vi "LinearPos Restrictions.vi"(5 "Robot Width":dbl, 6 "Robot Height":dbl, 7 "Pole Height \n(from ground)":dbl, 8 "Forearm Length":dbl, 9 "Backarm Length":dbl, 10 "newY":dbl, 11 "newX":dbl) -> (2 "modified Y":dbl, 3 "modified X":dbl)   [LabVIEW 2017]
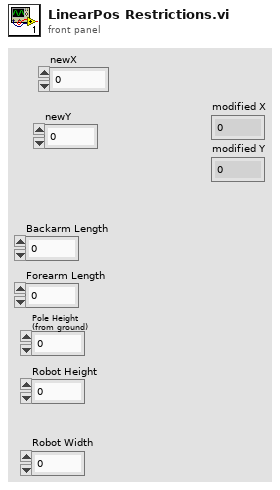
[diagram p1: front panel]
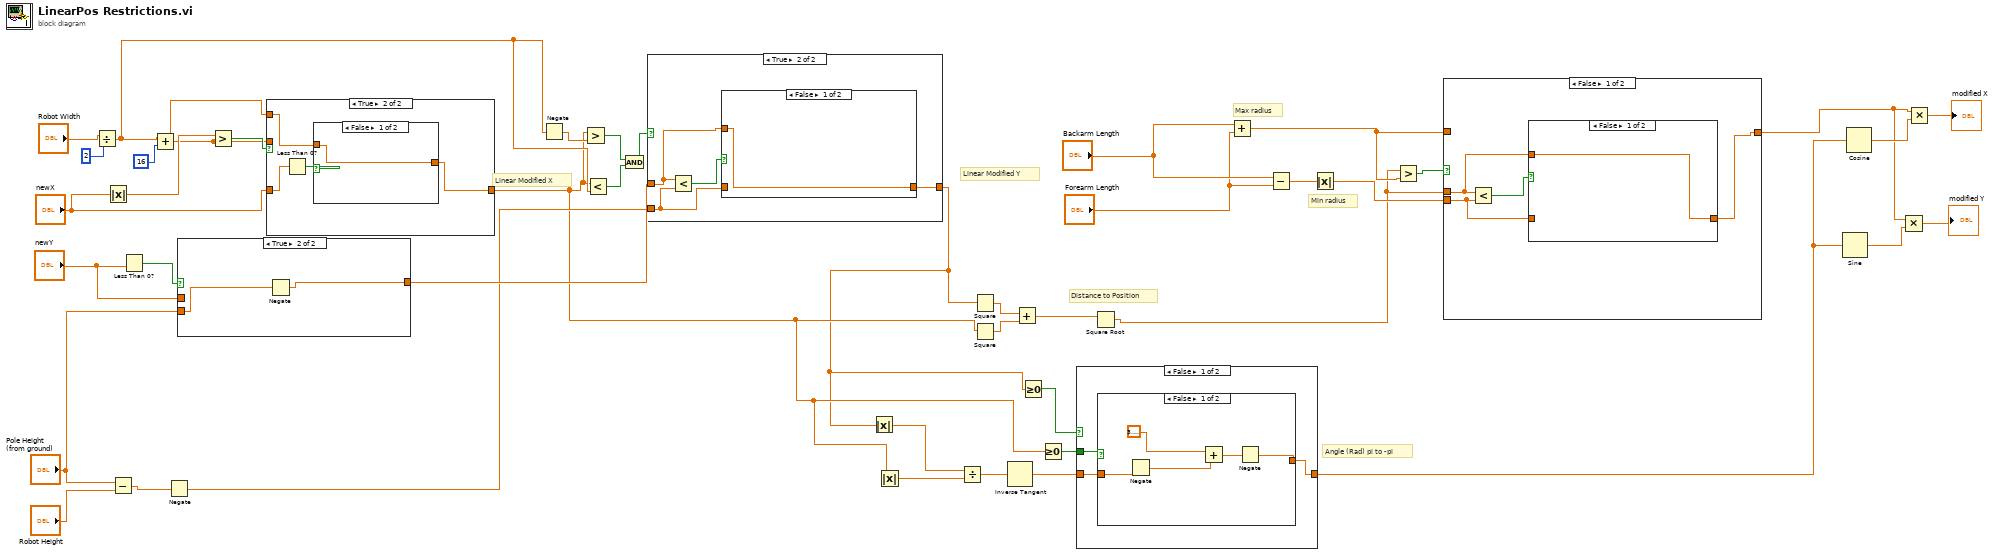
[diagram p0: block diagram]
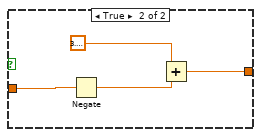
[diagram p4: hidden frame]
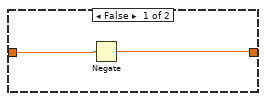
[diagram p6: hidden frame]
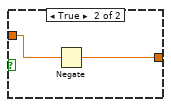
[diagram p11: hidden frame]
diagram:
  # "Min radius"
  # "Max radius"
  # "Angle (Rad) pi to -pi"
  # "Distance to Position"
  # "Linear Modified Y"
  # "Linear Modified X"
  n1 = Divide(x="Robot Width", y=2) -> (x/y=w35:dbl)
  n2 = Absolute Value(x="newX") -> (abs(x)=w39:dbl)
  n3 = Subtract(x="Pole Height \n(from ground)", y="Robot Height") -> (x-y=w26:dbl)
  n4 = Less Than 0?(x="newY") -> (x < 0?=w32:bool)
  n5 = Add(x=w35, y=16) -> (x+y=w37:dbl)
  n6 = Negate(x=w26) -> (-x=w25:dbl)
  n7 = case shown="True" w32 {
    tunnel: [w44 w45] -> w29
    tunnel: "newY" -> [w44 _]
    tunnel: "Pole Height \n(from ground)" -> [_ w46]
    frame False {
    }
    frame True {
      n8 = Negate(x=w46) -> (-x=w45:dbl)
    }
  }
  n9 = Greater?(x=w39, y=w37) -> (0:w40:bool)
  n10 = case shown="True" w40 {
    tunnel: w37 -> [_ _]
    tunnel: "newX" -> [w47 w51]
    tunnel: [w47 w48] -> w15
    tunnel: w37 -> [_ w49]
    frame False {
    }
    frame True {
      n11 = Less Than 0?(x=w51) -> (x < 0?=w50:bool)
      n12 = case shown="False" w50 {
        tunnel: w49 -> [w52 w54]
        tunnel: [w52 w53] -> w48
        frame False {
        }
        frame True {
          n13 = Negate(x=w54) -> (-x=w53:dbl)
        }
      }
    }
  }
  n14 = Negate(x=w35) -> (-x=w36:dbl)
  n15 = Greater?(x=w15, y=w36) -> (0:w34:bool)
  n16 = Less?(x=w15, y=w35) -> (x < y?=w33:bool)
  n17 = And(x=w34, y=w33) -> (x .and. y?=w30:bool)
  n18 = case shown="True" w30 {
    tunnel: w29 -> [w55 w57]
    tunnel: w25 -> [_ w58]
    tunnel: [w55 w56] -> w14
    frame False {
    }
    frame True {
      n19 = Less?(x=w57, y=w58) -> (x < y?=w59:bool)
      n20 = case shown="False" w59 {
        tunnel: w58 -> [_ w61]
        tunnel: [w60 w61] -> w56
        tunnel: w57 -> [w60 _]
        frame False {
        }
        frame True {
        }
      }
    }
  }
  n21 = Absolute Value(x=w14) -> (abs(x)=w21:dbl)
  n22 = Absolute Value(x=w15) -> (abs(x)=w20:dbl)
  n23 = Divide(x=w21, y=w20) -> (x/y=w19:dbl)
  n24 = Square(x=w14) -> (x^2=w24:dbl)
  n25 = Square(x=w15) -> (x^2=w23:dbl)
  n26 = Inverse Tangent(1:w19) -> (0:w16:dbl)
  n27 = Add(x=w24, y=w23) -> (x+y=w22:dbl)
  n28 = Greater Or Equal To 0?(x=w14) -> (x >= 0?=w18:bool)
  n29 = Greater Or Equal To 0?(x=w15) -> (x >= 0?=w17:bool)
  n30 = case shown="False" w18 {
    tunnel: w17 -> [w64 w76]
    tunnel: w16 -> [w63 w75]
    tunnel: [w62 w74] -> w6
    frame False {
      n31 = case shown="False" w64 {
        tunnel: w63 -> [w67 w73]
        tunnel: [w65 w70] -> w62
        frame False {
          n32 = Negate(x=w67) -> (-x=w69:dbl)
          n33 = Add(x=3.141592653589793, y=w69) -> (x+y=w66:dbl)
          n34 = Negate(x=w66) -> (-x=w65:dbl)
        }
        frame True {
          n35 = Negate(x=w73) -> (-x=w71:dbl)
          n36 = Add(x=3.141592653589793, y=w71) -> (x+y=w70:dbl)
        }
      }
    }
    frame True {
      n37 = case shown="True" w76 {
        tunnel: w75 -> [w78 w79]
        tunnel: [w77 w79] -> w74
        frame False {
          n38 = Negate(x=w78) -> (-x=w77:dbl)
        }
        frame True {
        }
      }
    }
  }
  n39 = Square Root(x=w22) -> (sqrt(x)=w7:dbl)
  n40 = Add(x="Backarm Length", y="Forearm Length") -> (x+y=w9:dbl)
  n41 = Subtract(x="Backarm Length", y="Forearm Length") -> (x-y=w11:dbl)
  n42 = Absolute Value(x=w11) -> (abs(x)=w8:dbl)
  n43 = Greater?(x=w7, y=w9) -> (0:w10:bool)
  n44 = case shown="False" w10 {
    tunnel: [w81 w86] -> w4
    tunnel: w9 -> [_ w86]
    tunnel: w8 -> [w82 _]
    tunnel: w7 -> [w80 _]
    frame False {
      n45 = Less?(x=w80, y=w82) -> (x < y?=w83:bool)
      n46 = case shown="False" w83 {
        tunnel: w82 -> [_ w85]
        tunnel: [w84 w85] -> w81
        tunnel: w80 -> [w84 _]
        frame False {
        }
        frame True {
        }
      }
    }
    frame True {
    }
  }
  n47 = Sine(x=w6) -> (sin(x)=w3:dbl)
  n48 = Cosine(x=w6) -> (cos(x)=w5:dbl)
  n49 = Multiply(x=w4, y=w3) -> (x*y=→"modified Y":dbl)
  n50 = Multiply(x=w4, y=w5) -> (x*y=→"modified X":dbl)
